vi "D触发器逻辑功能测试.vi"(6 "R`":bool, 7 "S`":bool, 9 "cp":bool, 10 "D":bool) -> (1 "Q`":bool, 2 "Q":bool)   [LabVIEW 2018]
panel:
  in  "结束":bool
  # "上升沿D触发器"
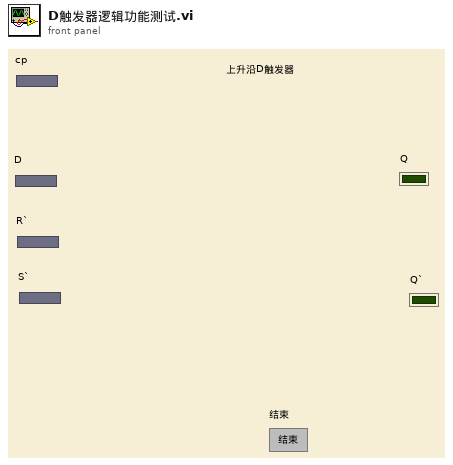
[diagram p1: front panel]
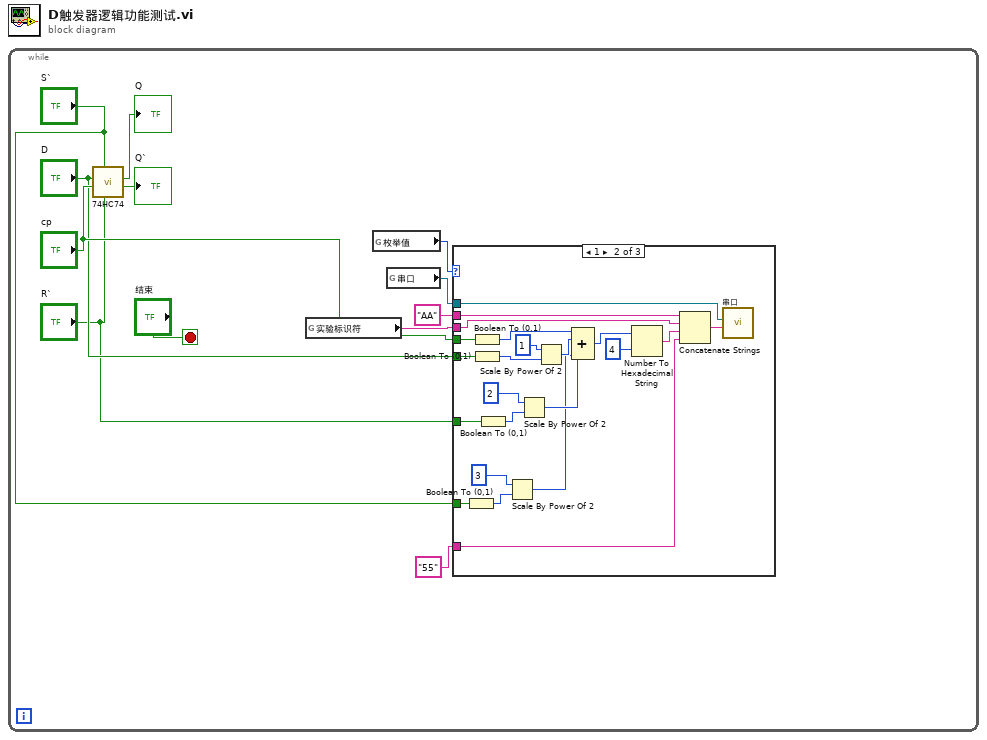
[diagram p0: block diagram]
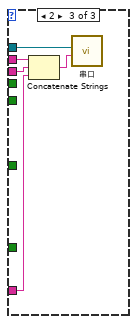
[diagram p3: hidden frame]
diagram:
  n1 = while {
    stop <- "结束" stop-if-true
    n2 = call "74HC74.vi"("R`"="R`", "S`"="S`", "cp"="cp", "D"="D") -> ("Q`"=→"Q`":bool, "Q"=→"Q":bool)  [unwired: 6 in]
    n3 = global read "全局变量.vi" "实验标识符"() -> (w7:string)
    n4 = global read "全局变量.vi" "枚举值"() -> (w9:i8)
    n5 = global read "全局变量.vi" "串口"() -> (w8:refnum<visa-resource-name>)
    n6 = case shown="1" w9 {
      tunnel: "cp" -> [_ w29 _]
      tunnel: w8 -> [_ w28 w37]
      tunnel: w7 -> [_ w27 w38]
      tunnel: "55" -> [_ w26 w35]
      tunnel: "AA" -> [_ w25 w36]
      tunnel: "D" -> [_ w15 _]
      tunnel: "R`" -> [_ w14 _]
      tunnel: "S`" -> [_ w13 _]
      frame 0, Default {
      }
      frame 1 {
        n7 = Boolean To (0,1)(Boolean=w13) -> (0, 1=w18:i16)
        n8 = Boolean To (0,1)(Boolean=w29) -> (0, 1=w33:i16)
        n9 = Boolean To (0,1)(Boolean=w15) -> (0, 1=w31:i16)
        n10 = Boolean To (0,1)(Boolean=w14) -> (0, 1=w20:i16)
        n11 = Scale By Power Of 2(n=3, x=w18) -> (x*2^n=w16:i16)
        n12 = Scale By Power Of 2(n=2, x=w20) -> (x*2^n=w21:i16)
        n13 = Scale By Power Of 2(n=1, x=w31) -> (x*2^n=w32:i16)
        n14 = Compound Arithmetic op=ADD ("复合运算")(w33, w32, w21, w16) -> (w24:i16)
        n15 = Number To Hexadecimal String(1:4, 2:w24) -> (0:w22:string)
        n16 = Concatenate Strings(w25, w27, w22, w26) -> (w34:string)
        n17 = call "串口.vi"("字符串"=w34, "VISA resource name"=w28) -> ()  [unwired: 10 in]
      }
      frame 2 {
        n18 = Concatenate Strings(w36, w38, w35) -> (w39:string)
        n19 = call "串口.vi"("字符串"=w39, "VISA resource name"=w37) -> ()  [unwired: 10 in]
      }
    }
  }
